vi "Initialize.vi"(8 "error in (no error)":errorcluster, 9 "Picture Control Ref":refnum<vi>, 10 "Path Control Ref":refnum<vi>, 11 "Reference Control in":refnum<class "Reference Control.lvclass">) -> (0 "error out":errorcluster, 3 "Reference Control out":refnum<class "Reference Control.lvclass">)   [LabVIEW 2016, in "Reference Control.lvclass"]
uses:
  Reference Control.lvclass
  Reference Control.lvclass/Reference Control.ctl
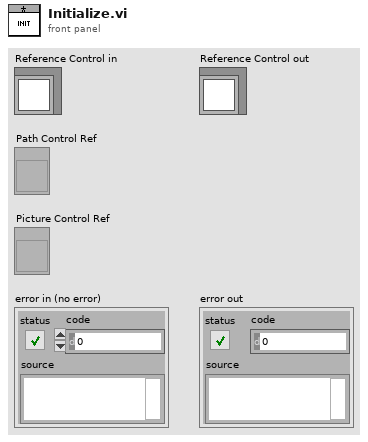
[diagram p1: front panel]
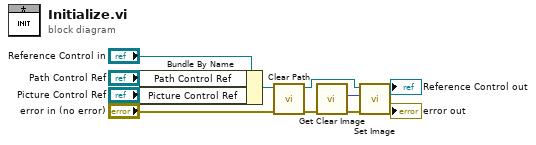
[diagram p0: block diagram]
diagram:
  n1 = Bundle By Name(cluster="Reference Control in", "Path Control Ref"="Path Control Ref", "Picture Control Ref"="Picture Control Ref") -> (w8:refnum<class "Reference Control.lvclass">)
  n2 = call "Clear Path.vi"("error in (no error)"="error in (no error)", "Reference Control in"=w8) -> ("error out"=w11:errorcluster, "Reference Control out"=w9:refnum<class "Reference Control.lvclass">)  [unwired: 8 in]
  n3 = call "Get Clear Image.vi"("error in (no error)"=w11) -> ("error out"=w4:errorcluster, "Picture"=w5:picture)  [unwired: 9 in]
  n4 = call "Set Image.vi"("error in (no error)"=w4, "Picture"=w5, "Reference Control in"=w9) -> ("error out"=→"error out":errorcluster, "Reference Control out"=→"Reference Control out":refnum<class "Reference Control.lvclass">)  [unwired: 7 in]
